vi "Replicate_Build_Specs_and_Compile.vi"() -> ()   [LabVIEW 2021]
panel:
  out "error out":errorcluster
  in  "Build Spec to Replicate":string="mmWave Demodulator(FPGA)"
  in  "Number of Build Specs to create":i32
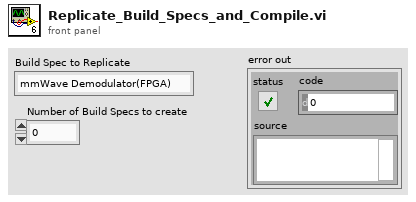
[diagram p1: front panel]
types:
  T1 = cluster{"ProjectPath":path, "TargetName":string, "BuildSpecName":string, "Build Specifications":refnum<vi>}[]
  T2 = cluster{"ProjectPath":path, "TargetName":string, "BuildSpecName":string, "Build Specifications":refnum<vi>}
  T3 = typedef "niFpgaBuild_BuildSpecPath.ctl" = cluster{"ProjectPath":path, "TargetName":string, "BuildSpecName":string}
  T4 = typedef "niFpgaBuild_JobState.ctl" = enum16{"Waiting", "Working", "Cancelled", "Complete", "Error"}
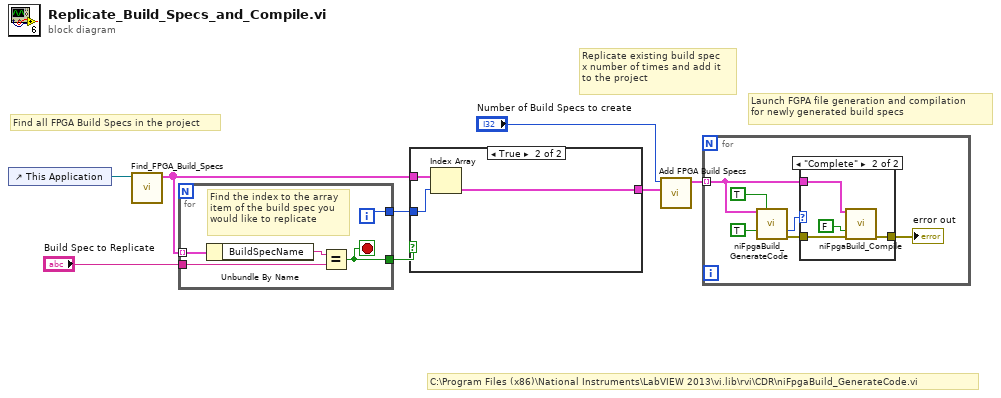
[diagram p0: block diagram]
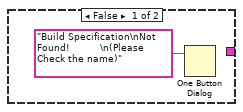
[diagram p3: hidden frame]
diagram:
  # "C:\\Program Files (x86)\\National Instruments\\LabVIEW 2013\\vi.lib\\rvi\\CDR\\niFpgaBuild_GenerateCode.vi"
  # "Launch FGPA file generation and compilation\nfor newly generated build specs"
  # "Replicate existing build spec\nx number of times and add it\nto the project"
  # "Find all FPGA Build Specs in the project"
  n1 = control-ref of="This Application"() -> (w8:refnum<vi>)
  n2 = call "Find_FPGA_Build_Specs.vi"("Application in"=w8) -> ("Build Spec Details"=w5:T1)  [unwired: 10 in]
  n3 = for {
    tunnel: w5 -> [w13] mode=indexing
    tunnel: "Build Spec to Replicate" -> [w11]
    tunnel: [w10] -> w4
    tunnel: [w9] -> w6
    i -> [w10]
    stop <- w9 stop-if-true
    # "Find the index to the array\nitem of the build spec you\nwould like to replicate"
    n4 = Unbundle By Name(w13) -> ("BuildSpecName"=w12:string)
    n5 = Equal?(x=w12, y=w11) -> (x = y?=w9:bool)
  }
  n6 = case shown="True" w6 {
    tunnel: w5 -> [_ w17]
    tunnel: w4 -> [_ w16]
    tunnel: [_ w15] -> w3
    frame False {
      n7 = One Button Dialog(message="Build Specification\nNot Found!          \n(Please Check the name)") -> ()  [unwired: 1 in, 1 out]
    }
    frame True {
      n8 = Index Array(array=w17, index=w16) -> (element=w15:T2)
    }
  }
  n9 = call "Add FPGA Build Specs.vi"("build spec details"=w3, "Number of Build Specs"="Number of Build Specs to create") -> ("Added Build Specs"=w1:T3[])  [unwired: 9 in]
  n10 = for {
    tunnel: w1 -> [w18] mode=indexing
    n11 = call <vilib>:"niFpgaBuild_GenerateCode.vi"("build spec path"=w18, "display status dialogs(T)"=TRUE, "wait until done"=TRUE) -> ("state"=w22:T4, "error out"=w21:errorcluster)  [unwired: 11 in]
    n12 = case shown="\"Complete\"" w22 {
      tunnel: w21 -> [w24 w28]
      tunnel: w18 -> [_ w27]
      tunnel: [w24 w26] -> w20
      frame Default {
      }
      frame "Complete" {
        n13 = call <vilib>:"niFpgaBuild_Compile.vi"("build spec path"=w27, "wait until done"=FALSE, "error in (no error)"=w28) -> ("error out"=w26:errorcluster)  [unwired: 11 in, 1 out]
      }
    }
    "error out" <- w20
  }
